vi "Demarcate.vi"(7 "Mode":enum16{"Read", "Write"}(ring)=enum."Write", 8 "error in":errorcluster, 10 "工位二扭矩偏移":cluster{"正向":dbl, "逆向":dbl}, 11 "工位一扭矩偏移":cluster{"正向":dbl, "逆向":dbl}) -> (0 "error out":errorcluster, 3 "Sensor OUT":T1)   [LabVIEW 2020]
panel:
  out "工位二扭矩偏移":cluster{"正向":dbl, "逆向":dbl}
  out "工位一扭矩偏移":cluster{"正向":dbl, "逆向":dbl}
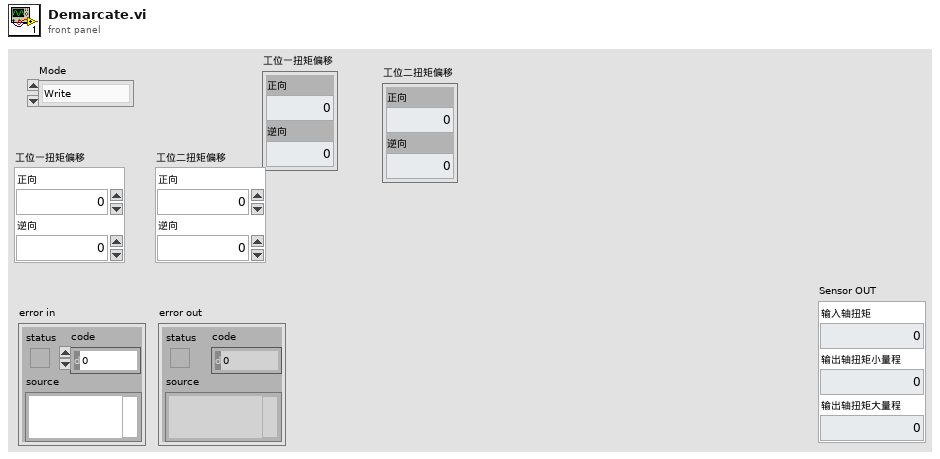
[diagram p1: front panel]
types:
  T1 = cluster{"输入轴扭矩":dbl, "输出轴扭矩小量程":dbl, "输出轴扭矩大量程":dbl}
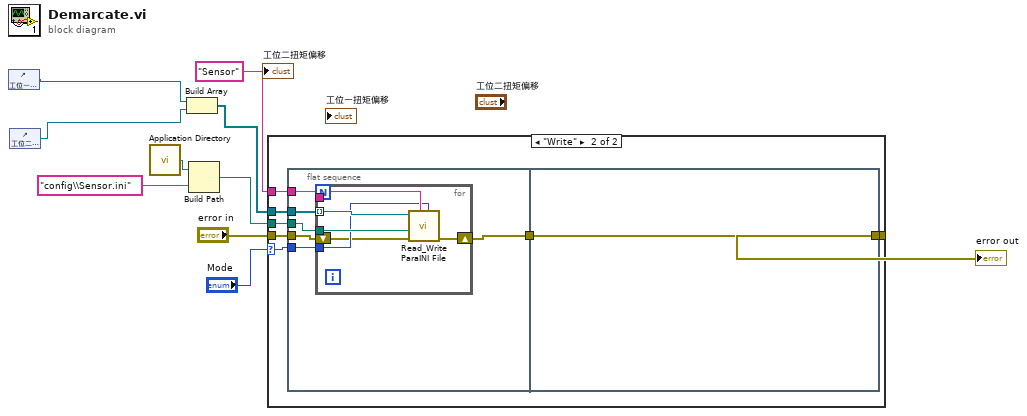
[diagram p0: block diagram]
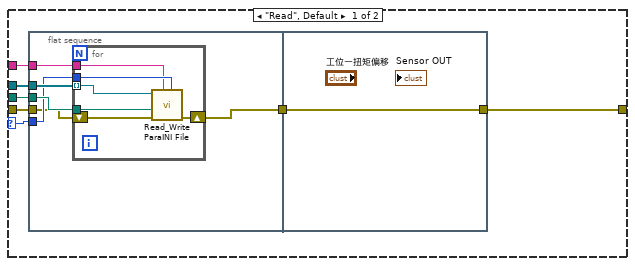
[diagram p2: hidden frame]
diagram:
  n1 = control-ref of="工位一扭矩偏移"() -> (w2:refnum<vi>)
  n2 = control-ref of="工位二扭矩偏移"() -> (w1:refnum<vi>)
  n3 = call <vilib>:"Application Directory.vi"() -> ("Application Directory"=w9:path)
  n4 = Build Array(w2, w1) -> (w3:refnum<vi>[])
  n5 = Build Path(base path=w9, name or relative path="config\\Sensor.ini" ("名称或相对路径")) -> (appended path=w7:path)
  n6 = case shown="\"Write\"" "Mode" {
    selector: "Mode" -> [w15 w34]
    tunnel: w3 -> [w16 w37]
    tunnel: "Sensor" ("Section") -> [w14 w36]
    tunnel: w7 -> [w17 w35]
    tunnel: "error in" -> [w13 w33]
    tunnel: [w12 w32] -> w4
    frame "Read", Default {
      n7 = flat-sequence {
        tunnel: w17 -> [w23]
        tunnel: w16 -> [w22]
        tunnel: w15 -> [w21]
        tunnel: w14 -> [w20]
        tunnel: w13 -> [w19]
        tunnel: [w18] -> w11
        tunnel: [w30] -> w12
        tunnel: w11 -> [w30]
        frame #0 {
          n8 = for {
            tunnel: w23 -> [w29]
            tunnel: w22 -> [w28] mode=indexing
            tunnel: w21 -> [w27]
            tunnel: w20 -> [w26]
            shift-right: [w24] -> w18
            shift-left: w19 -> [w25]
            n9 = call "Read_Write ParaINI File.vi"("Mode"=w27, "Section"=w26, "error in"=w25, "Filepath"=w29, "Ctl Refnum"=w28) -> ("error out"=w24:errorcluster)  [unwired: 6 in]
          }
        }
        frame #1 {
        }
      }
    }
    frame "Write" {
      n10 = flat-sequence {
        tunnel: w37 -> [w43]
        tunnel: w36 -> [w42]
        tunnel: w35 -> [w41]
        tunnel: w34 -> [w40]
        tunnel: w33 -> [w39]
        tunnel: [w38] -> w31
        tunnel: [w50] -> w32
        tunnel: w31 -> [w50]
        frame #0 {
          n11 = for {
            tunnel: w43 -> [w49] mode=indexing
            tunnel: w42 -> [w48]
            tunnel: w41 -> [w47]
            tunnel: w40 -> [w46]
            shift-right: [w44] -> w38
            shift-left: w39 -> [w45]
            n12 = call "Read_Write ParaINI File.vi"("Mode"=w46, "Section"=w48, "error in"=w45, "Filepath"=w47, "Ctl Refnum"=w49) -> ("error out"=w44:errorcluster)  [unwired: 6 in]
          }
        }
        frame #1 {
        }
      }
    }
  }
  "error out" <- w4
